vi "Board Info Report.vi"(8 "error in (no error)":errorcluster) -> (0 "error out":errorcluster, 3 "Report":string)   [LabVIEW 2022 SP3]
uses:
  <vilib>/Instr/_visa.llb/VISA Flush IO Buffer Mask.ctl
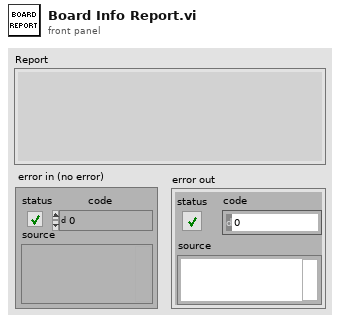
[diagram p1: front panel]
types:
  T1 = typedef "VISA Flush IO Buffer Mask.ctl" = u16
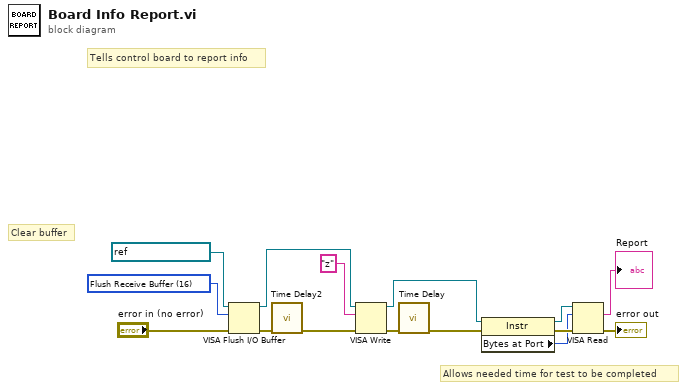
[diagram p0: block diagram]
diagram:
  w14 = T1 16 items=["Flush Receive Buffer"=16, "Write Transmit Buffer to Device"=32, "Flush Receive Buffer (No I/O)"=64, "Flush Transmit Buffer"=128] ("Mask")
  # "Allows needed time for test to be completed"
  # "Tells control board to report info"
  # "Clear buffer"
  n1 = VISA Flush I/O Buffer(VISA resource name=refnum<visa-resource-name> "ControlBoard", mask (16)=w14, error in (no error)="error in (no error)") -> (VISA resource name out=w12:refnum<visa-resource-name>, error out=w9:errorcluster)
  n2 = call "Time Delay2"("error in (no error)"=w9) -> ("error out"=w8:errorcluster)  [unwired: 10 in]
  n3 = VISA Write(VISA resource name=w12, write buffer="z", error in (no error)=w8) -> (VISA resource name out=w6:refnum<visa-resource-name>, error out=w13:errorcluster)  [unwired: 1 out]
  n4 = call "Time Delay"("error in (no error)"=w13) -> ("error out"=w7:errorcluster)  [unwired: 10 in]
  n5 = property class="Instr"(reference=w6, error in=w7) -> (reference out=w5:refnum<visa-resource-name>, error out=w4:errorcluster, "Bytes at Port"=w3:u32)
  n6 = VISA Read(VISA resource name=w5, byte count=w3, error in (no error)=w4) -> (read buffer=→"Report":string, error out=→"error out":errorcluster)  [unwired: 2 out]
